vi "SaveGestures.vi"(10 "error in (no error)":errorcluster, 11 ".NET Refnum in":refnum<k24>) -> (2 "error out":errorcluster, 3 "All Gestures":cluster{T1[], T6[], T7[], T8[]})   [LabVIEW 2010, in "lvleap.lvlib"]
uses:
  lvleap.lvlib
  C:/Users/mraj/Desktop/src/Libs/LeapCSharp.NET3.5.dll
  Libs/LeapCSharp.NET3.5.dll
  Controls/Gesture Swipe.ctl
  Controls/Gesture Common.ctl
  Controls/Gesture Type.ctl
  Controls/Gesture State.ctl
  Controls/Vector.ctl
  Controls/Gesture Circle.ctl
  Controls/Gesture Screen Tap.ctl
  Controls/Gesture Key Tap.ctl
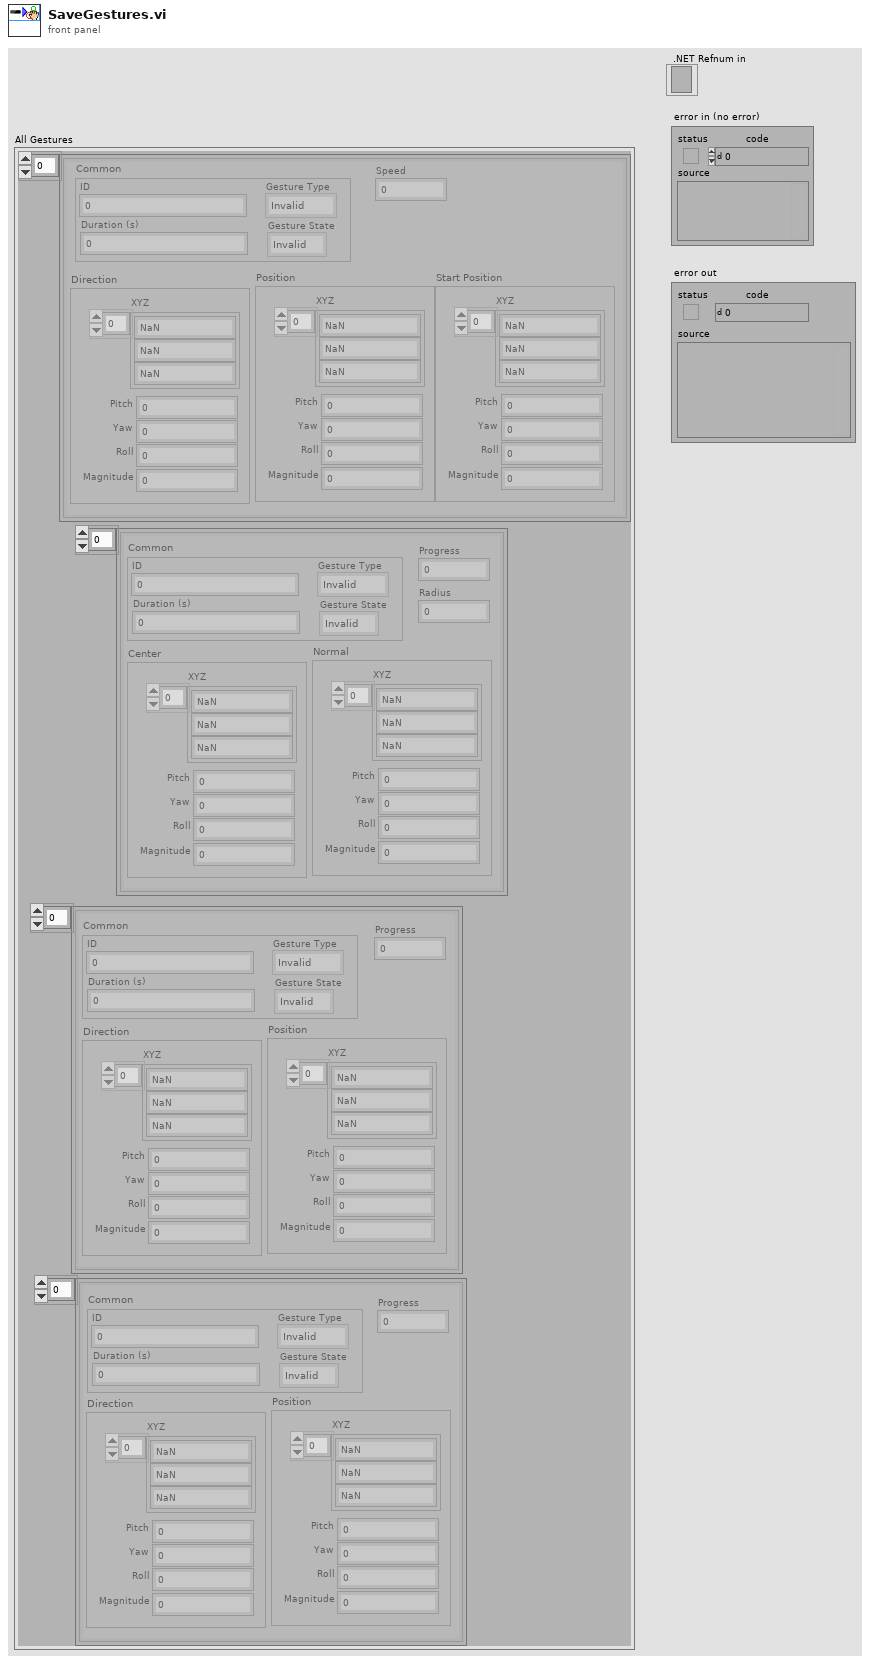
[diagram p1: front panel]
types:
  T1 = typedef "lvleap.lvlib/Gesture Swipe.ctl" = cluster{"Common":T2, "Direction":T5, "Position":T5, "Start Position":T5, "Speed":dbl}
  T2 = typedef "lvleap.lvlib/Gesture Common.ctl" = cluster{"ID":i32, "Duration (s)":dbl, "Gesture Type":T3, "Gesture State":T4}
  T3 = typedef "lvleap.lvlib/Gesture Type.ctl" = enum16{"Invalid", "Swipe", "Circle", "Screen Tap", "Key Tap"}
  T4 = typedef "lvleap.lvlib/Gesture State.ctl" = enum16{"Invalid", "Start", "Update", "Stop"}
  T5 = typedef "lvleap.lvlib/Vector.ctl" = cluster{"Pitch":sgl, "Yaw":sgl, "Roll":sgl, "Magnitude":sgl, "XYZ":sgl[]}
  T6 = typedef "lvleap.lvlib/Gesture Circle.ctl" = cluster{"Common":T2, "Center":T5, "Normal":T5, "Progress":dbl, "Radius":dbl}
  T7 = typedef "lvleap.lvlib/Gesture Screen Tap.ctl" = cluster{"Common":T2, "Direction":T5, "Position":T5, "Progress":dbl}
  T8 = typedef "lvleap.lvlib/Gesture Key Tap.ctl" = cluster{"Common":T2, "Direction":T5, "Position":T5, "Progress":dbl}
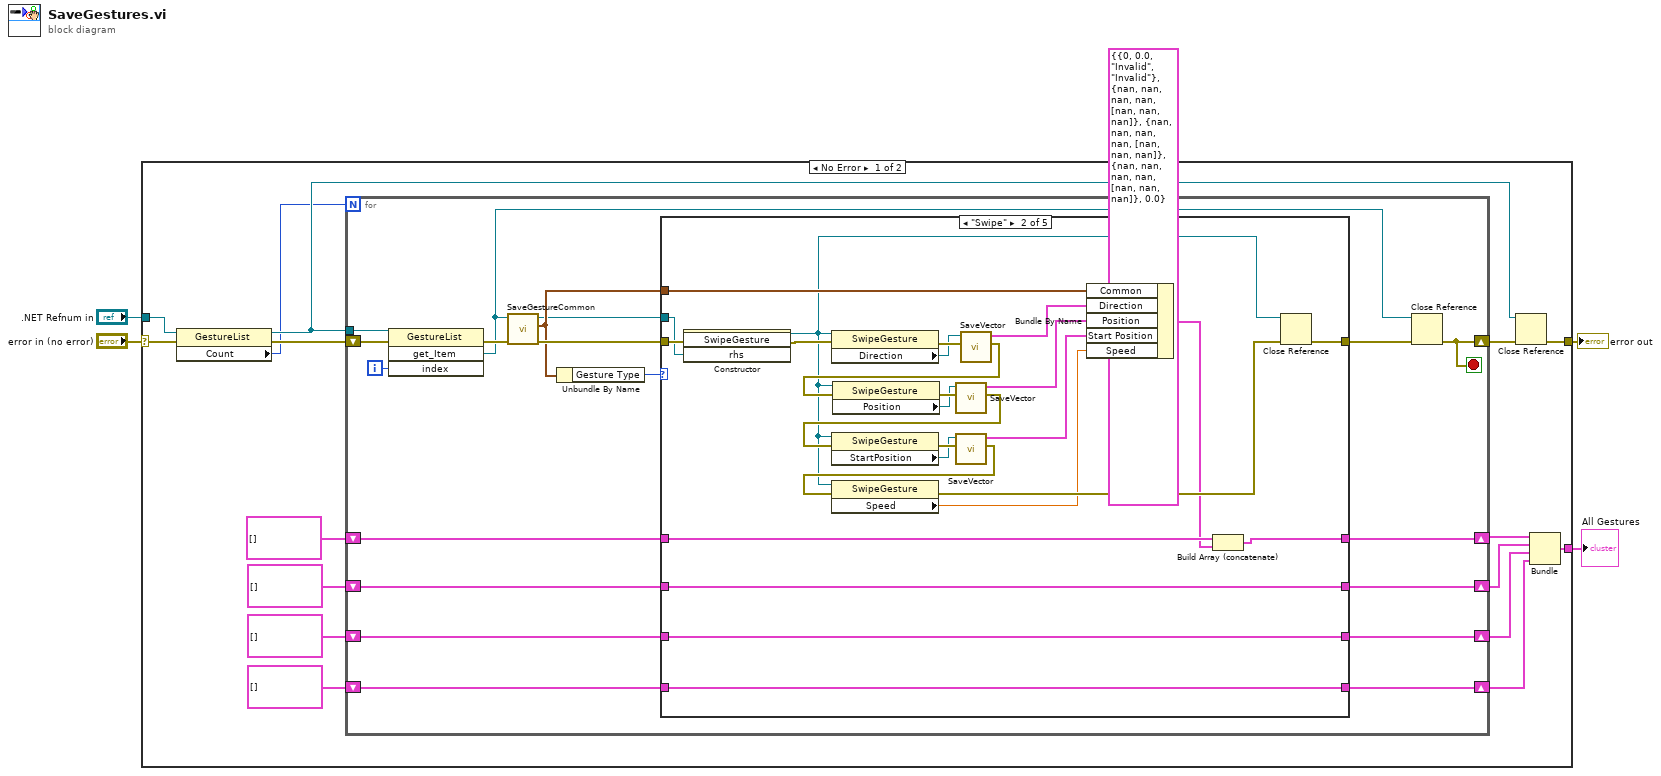
[diagram p0: block diagram]
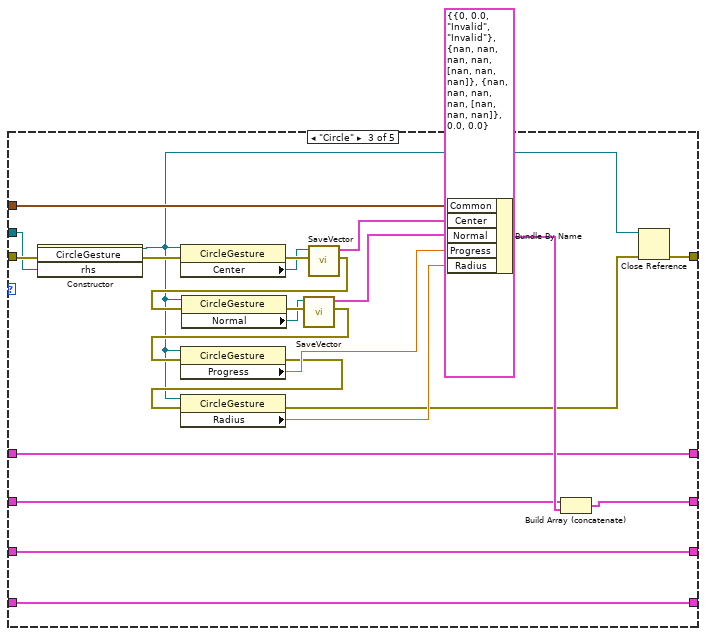
[diagram p3: hidden frame]
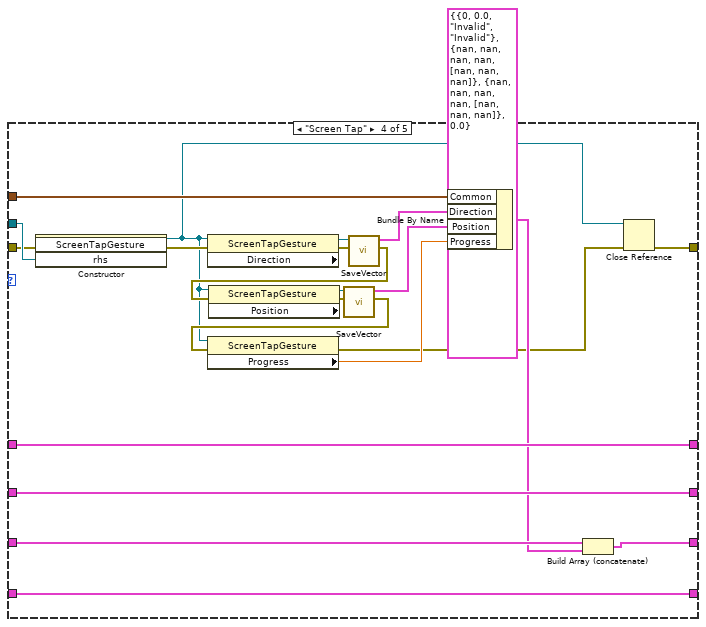
[diagram p4: hidden frame]
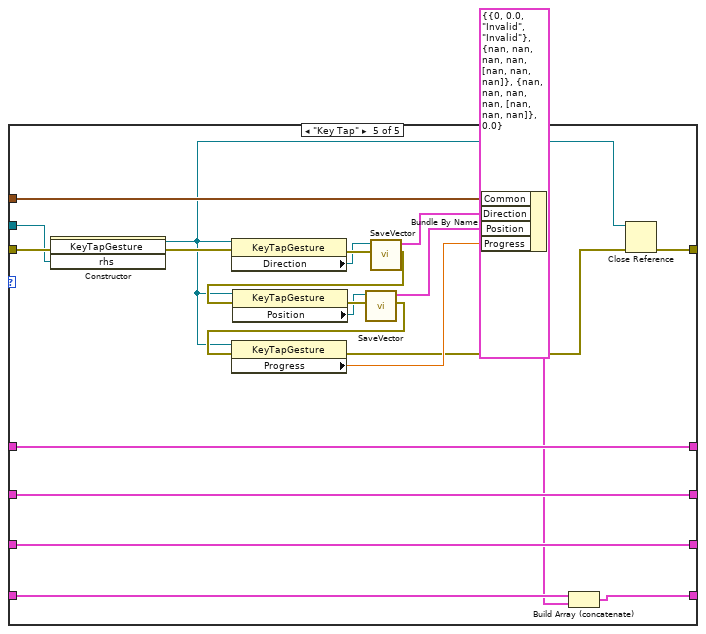
[diagram p5: hidden frame]
diagram:
  n1 = case shown="No Error" "error in (no error)" {
    selector: "error in (no error)" -> [w17 w143]
    tunnel: ".NET Refnum in" -> [w18 _]
    tunnel: [w15 w143] -> w3
    tunnel: [w5 _] -> w1
    frame No Error {
      n2 = property class="GestureList"(reference=w18, error in=w17) -> (reference out=w19:refnum<k24>, error out=w20:errorcluster, "Count"=w14:i32)
      n3 = for {
        N: w14 -> [_]
        tunnel: w19 -> [w37]
        shift-right: [w35] -> w16
        shift-left: w20 -> [w38]
        shift-right: [w29] -> w9
        shift-left: T1[] [] -> [w30]
        shift-right: [w27] -> w8
        shift-left: T6[] [] -> [w28]
        shift-right: [w25] -> w7
        shift-left: T7[] [] -> [w26]
        shift-right: [w23] -> w6
        shift-left: T8[] [] -> [w24]
        i -> [w36]
        stop <- w35 stop-if-true
        n4 = invoke class="GestureList" method="get_Item"(reference=w37, error in=w38, "index"=w36) -> (error out=w39:errorcluster, "get_Item"=w22:refnum<k24>)  [unwired: 1 in, 2 out]
        n5 = call "SaveGestureCommon.vi"("error in (no error)"=w39, ".NET Refnum in"=w22) -> ("error out"=w34:errorcluster, "Gesture Common"=w31:T2, ".NET Refnum Passthrough"=w21:refnum<k24>)  [unwired: 7 in]
        n6 = Unbundle By Name(w31) -> ("Gesture Type"=w33:T3)
        n7 = case shown="\"Swipe\"" w33 {
          tunnel: w21 -> [_ w47 w76 w102 w120]
          tunnel: w34 -> [w44 w49 w77 w101 w125]
          tunnel: [w44 w46 w74 w99 w123] -> w32
          tunnel: w31 -> [_ w69 w96 w119 w142]
          tunnel: w30 -> [w43 w55 w80 w109 w132]
          tunnel: [w43 w53 w80 w109 w132] -> w29
          tunnel: w28 -> [w42 w52 w82 w107 w131]
          tunnel: [w42 w52 w81 w107 w131] -> w27
          tunnel: w26 -> [w41 w51 w79 w106 w130]
          tunnel: [w41 w51 w79 w104 w130] -> w25
          tunnel: w24 -> [w40 w50 w78 w103 w128]
          tunnel: [w40 w50 w78 w103 w126] -> w23
          frame "Invalid", Default {
          }
          frame "Swipe" {
            n8 = constructor class="SwipeGesture"(error in=w49, "rhs"=w47) -> (reference out=w45:refnum<k24>, error out=w48:errorcluster)  [unwired: 2 in, 2 out]
            n9 = property class="SwipeGesture"(reference=w45, error in=w48) -> (error out=w68:errorcluster, "Direction"=w67:refnum<k24>)  [unwired: 1 out]
            n10 = call "SaveVector.vi"("error in (no error)"=w68, "Leap Vector"=w67) -> ("error out"=w66:errorcluster, "Vector"=w59:T5)  [unwired: 8 in]
            n11 = property class="SwipeGesture"(reference=w45, error in=w66) -> (error out=w65:errorcluster, "Position"=w64:refnum<k24>)  [unwired: 1 out]
            n12 = call "SaveVector.vi"("error in (no error)"=w65, "Leap Vector"=w64) -> ("error out"=w61:errorcluster, "Vector"=w58:T5)  [unwired: 8 in]
            n13 = property class="SwipeGesture"(reference=w45, error in=w61) -> (error out=w63:errorcluster, "StartPosition"=w62:refnum<k24>)  [unwired: 1 out]
            n14 = call "SaveVector.vi"("error in (no error)"=w63, "Leap Vector"=w62) -> ("error out"=w60:errorcluster, "Vector"=w57:T5)  [unwired: 8 in]
            n15 = property class="SwipeGesture"(reference=w45, error in=w60) -> (error out=w71:errorcluster, "Speed"=w56:sgl)  [unwired: 1 out]
            n16 = Bundle By Name(cluster=T1 {"Common"={"ID"=0, "Duration (s)"=0.0, "Gesture Type"=enum."Invalid", "Gesture State"=enum."Invalid"}, "Direction"={"Pitch"=nan, "Yaw"=nan, "Roll"=nan, "Magnitude"=nan, "XYZ"=[nan, nan, nan]}, "Position"={"Pitch"=nan, "Yaw"=nan, "Roll"=nan, "Magnitude"=nan, "XYZ"=[nan, nan, nan]}, "Start Position"={"Pitch"=nan, "Yaw"=nan, "Roll"=nan, "Magnitude"=nan, "XYZ"=[nan, nan, nan]}, "Speed"=0.0} ("Gesture Swipe"), "Common"=w69, "Direction"=w59, "Position"=w58, "Start Position"=w57, "Speed"=w56) -> (w54:T1)
            n17 = Build Array (concatenate)(w55, w54) -> (w53:T1[])
            n18 = Close Reference(reference=w45, error in (no error)=w71) -> (error out=w46:errorcluster)
          }
          frame "Circle" {
            n19 = constructor class="CircleGesture"(error in=w77, "rhs"=w76) -> (reference out=w72:refnum<k24>, error out=w75:errorcluster)  [unwired: 2 in, 2 out]
            n20 = property class="CircleGesture"(reference=w72, error in=w75) -> (error out=w95:errorcluster, "Center"=w94:refnum<k24>)  [unwired: 1 out]
            n21 = call "SaveVector.vi"("error in (no error)"=w95, "Leap Vector"=w94) -> ("error out"=w93:errorcluster, "Vector"=w89:T5)  [unwired: 8 in]
            n22 = property class="CircleGesture"(reference=w72, error in=w93) -> (error out=w92:errorcluster, "Normal"=w91:refnum<k24>)  [unwired: 1 out]
            n23 = call "SaveVector.vi"("error in (no error)"=w92, "Leap Vector"=w91) -> ("error out"=w90:errorcluster, "Vector"=w88:T5)  [unwired: 8 in]
            n24 = property class="CircleGesture"(reference=w72, error in=w90) -> (error out=w83:errorcluster, "Progress"=w84:sgl)  [unwired: 1 out]
            n25 = property class="CircleGesture"(reference=w72, error in=w83) -> (error out=w73:errorcluster, "Radius"=w87:sgl)  [unwired: 1 out]
            n26 = Bundle By Name(cluster=T6 {"Common"={"ID"=0, "Duration (s)"=0.0, "Gesture Type"=enum."Invalid", "Gesture State"=enum."Invalid"}, "Center"={"Pitch"=nan, "Yaw"=nan, "Roll"=nan, "Magnitude"=nan, "XYZ"=[nan, nan, nan]}, "Normal"={"Pitch"=nan, "Yaw"=nan, "Roll"=nan, "Magnitude"=nan, "XYZ"=[nan, nan, nan]}, "Progress"=0.0, "Radius"=0.0} ("Gesture Circle"), "Common"=w96, "Center"=w89, "Normal"=w88, "Progress"=w84, "Radius"=w87) -> (w86:T6)
            n27 = Build Array (concatenate)(w82, w86) -> (w81:T6[])
            n28 = Close Reference(reference=w72, error in (no error)=w73) -> (error out=w74:errorcluster)
          }
          frame "Screen Tap" {
            n29 = constructor class="ScreenTapGesture"(error in=w101, "rhs"=w102) -> (reference out=w97:refnum<k24>, error out=w100:errorcluster)  [unwired: 2 in, 2 out]
            n30 = property class="ScreenTapGesture"(reference=w97, error in=w100) -> (error out=w118:errorcluster, "Direction"=w117:refnum<k24>)  [unwired: 1 out]
            n31 = call "SaveVector.vi"("error in (no error)"=w118, "Leap Vector"=w117) -> ("error out"=w116:errorcluster, "Vector"=w112:T5)  [unwired: 8 in]
            n32 = property class="ScreenTapGesture"(reference=w97, error in=w116) -> (error out=w115:errorcluster, "Position"=w114:refnum<k24>)  [unwired: 1 out]
            n33 = call "SaveVector.vi"("error in (no error)"=w115, "Leap Vector"=w114) -> ("error out"=w113:errorcluster, "Vector"=w111:T5)  [unwired: 8 in]
            n34 = property class="ScreenTapGesture"(reference=w97, error in=w113) -> (error out=w98:errorcluster, "Progress"=w110:sgl)  [unwired: 1 out]
            n35 = Bundle By Name(cluster=T7 {"Common"={"ID"=0, "Duration (s)"=0.0, "Gesture Type"=enum."Invalid", "Gesture State"=enum."Invalid"}, "Direction"={"Pitch"=nan, "Yaw"=nan, "Roll"=nan, "Magnitude"=nan, "XYZ"=[nan, nan, nan]}, "Position"={"Pitch"=nan, "Yaw"=nan, "Roll"=nan, "Magnitude"=nan, "XYZ"=[nan, nan, nan]}, "Progress"=0.0} ("Gesture Screen Tap"), "Common"=w119, "Direction"=w112, "Position"=w111, "Progress"=w110) -> (w105:T7)
            n36 = Build Array (concatenate)(w106, w105) -> (w104:T7[])
            n37 = Close Reference(reference=w97, error in (no error)=w98) -> (error out=w99:errorcluster)
          }
          frame "Key Tap" {
            n38 = constructor class="KeyTapGesture"(error in=w125, "rhs"=w120) -> (reference out=w121:refnum<k24>, error out=w124:errorcluster)  [unwired: 2 in, 2 out]
            n39 = property class="KeyTapGesture"(reference=w121, error in=w124) -> (error out=w141:errorcluster, "Direction"=w140:refnum<k24>)  [unwired: 1 out]
            n40 = call "SaveVector.vi"("error in (no error)"=w141, "Leap Vector"=w140) -> ("error out"=w139:errorcluster, "Vector"=w135:T5)  [unwired: 8 in]
            n41 = property class="KeyTapGesture"(reference=w121, error in=w139) -> (error out=w138:errorcluster, "Position"=w137:refnum<k24>)  [unwired: 1 out]
            n42 = call "SaveVector.vi"("error in (no error)"=w138, "Leap Vector"=w137) -> ("error out"=w136:errorcluster, "Vector"=w134:T5)  [unwired: 8 in]
            n43 = property class="KeyTapGesture"(reference=w121, error in=w136) -> (error out=w122:errorcluster, "Progress"=w133:sgl)  [unwired: 1 out]
            n44 = Bundle By Name(cluster=T8 {"Common"={"ID"=0, "Duration (s)"=0.0, "Gesture Type"=enum."Invalid", "Gesture State"=enum."Invalid"}, "Direction"={"Pitch"=nan, "Yaw"=nan, "Roll"=nan, "Magnitude"=nan, "XYZ"=[nan, nan, nan]}, "Position"={"Pitch"=nan, "Yaw"=nan, "Roll"=nan, "Magnitude"=nan, "XYZ"=[nan, nan, nan]}, "Progress"=0.0} ("Gesture Key Tap"), "Common"=w142, "Direction"=w135, "Position"=w134, "Progress"=w133) -> (w127:T8)
            n45 = Build Array (concatenate)(w128, w127) -> (w126:T8[])
            n46 = Close Reference(reference=w121, error in (no error)=w122) -> (error out=w123:errorcluster)
          }
        }
        n47 = Close Reference(reference=w22, error in (no error)=w32) -> (error out=w35:errorcluster)
      }
      n48 = Close Reference(reference=w19, error in (no error)=w16) -> (error out=w15:errorcluster)
      n49 = Bundle(w9, w8, w7, w6) -> (w5:cluster{T1[], T6[], T7[], T8[]})  [unwired: 1 in]
    }
    frame Error {
    }
  }
  "error out" <- w3
  "All Gestures" <- w1
